vi "stop_stream_funcGlobal.vi"(10 "write?":bool=TRUE, 11 "queue out":refnum<queue>) -> (3 "queue out 2":refnum<queue>)   [LabVIEW 2015, in "lightfield_panel.lvclass"]
uses:
  lightfield_panel.lvclass
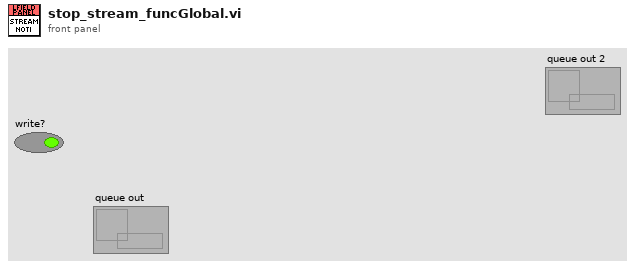
[diagram p1: front panel]
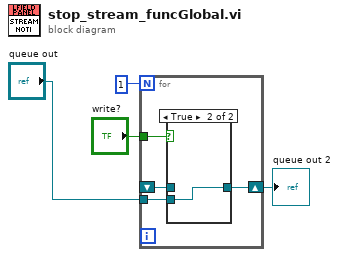
[diagram p0: block diagram]
diagram:
  n1 = for {
    N: 1 -> [_]
    tunnel: "write?" -> [w8]
    tunnel: "queue out" -> [w7]
    shift-right: [w6] -> w1
    shift-left: _ -> [w5]
    n2 = case shown="True" w8 {
      tunnel: w7 -> [_ w10]
      tunnel: [w9 w10] -> w6
      tunnel: w5 -> [w9 _]
      frame False {
      }
      frame True {
      }
    }
  }
  "queue out 2" <- w1
